vi "Build equal unit test strings.vi"(6 "String 2":string, 9 "String":string, 10 "Label":string, 11 "x+y":dbl) -> (1 "Chaîne 2":string, 2 "Chaîne":string, 3 "Chaîne 3":string, 4 "Numérique":i32)   [LabVIEW 2021]
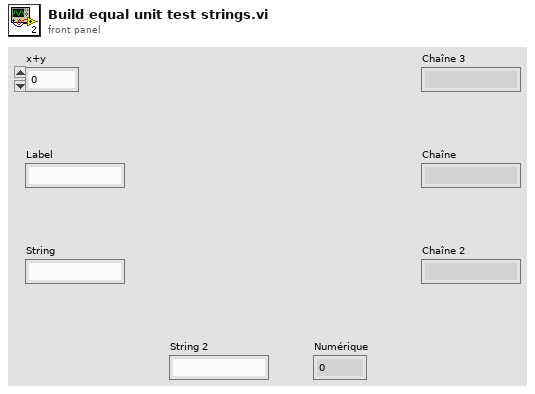
[diagram p1: front panel]
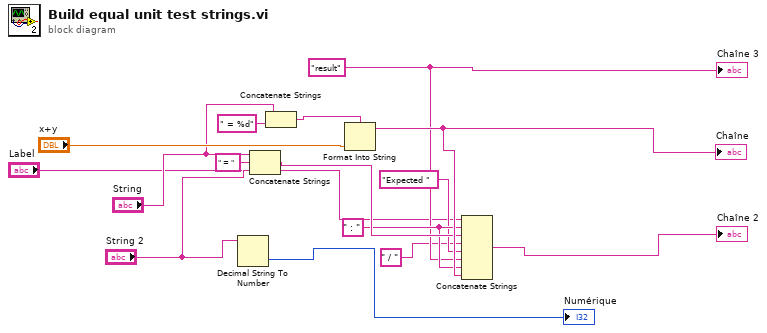
[diagram p0: block diagram]
diagram:
  w9 = " : " ("chaîne")
  w5 = "result"
  n1 = Decimal String To Number(string="String 2") -> (number=→"Numérique":i32)  [unwired: 2 in, 1 out]
  n2 = Concatenate Strings("String", " = " ("chaîne"), "String 2") -> (w10:string)
  n3 = Concatenate Strings("String", " = %d" ("chaîne")) -> (w13:string)
  n4 = Format Into String(format string=w13, "x+y") -> (resulting string=w14:string)  [unwired: 2 in, 1 out]
  "Chaîne" <- w14
  n5 = Concatenate Strings("Label", w9, w10, " / " ("chaîne"), "Expected " ("chaîne"), w5, w9, w14) -> (→"Chaîne 2":string)
  "Chaîne 3" <- w5
